vi "RichToFlatcif_manager_OrchReturn.vi"(5 "OutputClusterType":T1, 11 "InputCluster":T3) -> (3 "OutputCluster":T1)   [LabVIEW 2021, in "CIF_Manager_server.lvlib"]
uses:
  CIF_Manager_server.lvlib
  cif_manager_OrchReturn.ctl
  cif_common_Status.ctl
  cif_manager_OrchReturn_Flat.ctl
  cif_common_Status_Flat.ctl
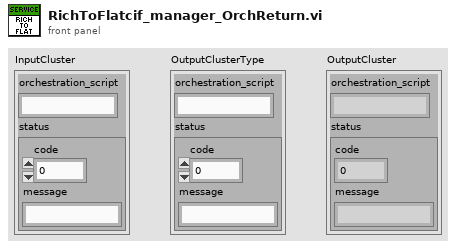
[diagram p1: front panel]
types:
  T1 = typedef "CIF_Manager_server.lvlib/cif_manager_OrchReturn_Flat.ctl" = cluster{"orchestration_script":string, "status":T2}
  T2 = typedef "CIF_Manager_server.lvlib/cif_common_Status_Flat.ctl" = cluster{"code":i32, "message":string}
  T3 = typedef "CIF_Manager_server.lvlib/cif_manager_OrchReturn.ctl" = cluster{"orchestration_script":string, "status":T4}
  T4 = typedef "CIF_Manager_server.lvlib/cif_common_Status.ctl" = cluster{"code":i32, "message":string}
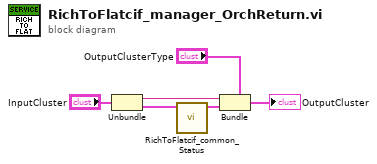
[diagram p0: block diagram]
diagram:
  n1 = Unbundle "Unbundle"("InputCluster") -> ("orchestration_script"=w3:string, "status"=w2:T4)
  n2 = call "RichToFlatcif_common_Status.vi"("InputCluster"=w2) -> ("OutputCluster"=w1:T2)  [unwired: 10 in]
  n3 = Bundle "Bundle"(cluster="OutputClusterType", "orchestration_script"=w3, "status"=w1) -> (→"OutputCluster":T1)
